vi "Get To Target Mock.vi"(0 "Encoder Right":dbl, 1 "Encoder Left":dbl, 2 "Robot Angle":dbl) -> (4 "Goal X":dbl, 5 "Left Motor":dbl, 6 "Position X":dbl, 7 "Position Y":dbl, 8 "Goal Y":dbl, 9 "Right Motor":dbl)   [LabVIEW 2016]
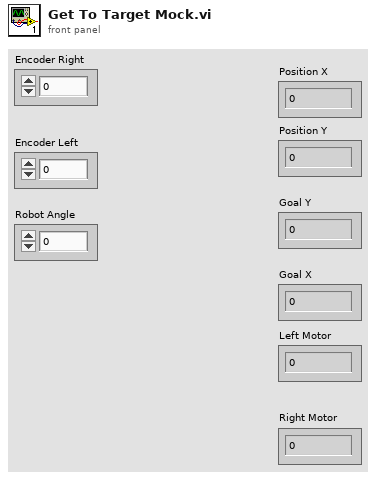
[diagram p1: front panel]
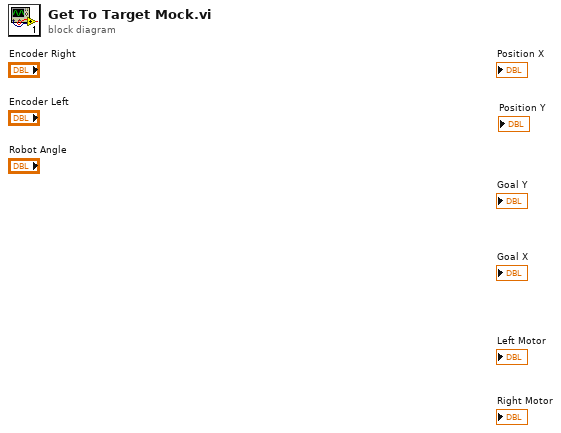
[diagram p0: block diagram]
diagram:
